vi "GameToIAStateDefensive.vi"(8 "error in (no error)":errorcluster, 11 "Game in":refnum<class "Game.lvclass">) -> (0 "error out":errorcluster, 2 "IA State out":T1={"our_robots"=[], "enemy_robots"=[], "balls"=[], "geometry"={"line_width"=0, "field_length"=0, "field_width"=0, "boundary_width"=0, "referee_width"=0, "goal_width"=0, "goal_depth"=0, "goal_wall_width"=0, "center_circle_radius"=0, "defense_radius"=0, "defense_stretch"=0, "free_kick_from_defense_dist"=0, "penalty_spot_from_field_line_dist"=0, "penalty_line_from_spot_dist"=0}, "IA Judge"={"stage"="", "command"="", "our_goalie_id"=0.0, "enemy_goalie_id"=0.0, "command enum"=enum."Halt", "Time"=enum."Azul", "Point"={"x"=0.0, "y"=0.0}}, "Received Timestamp"=timestamp(0 s since 1904-01-01), "Events"={"Touch"=FALSE, "Ball out"=FALSE, "id touch"=0.0, "Ball out of \nVision"=FALSE, "Ball inside \nGoalie area"=FALSE, "Robot not responding"=FALSE, "Robots responding status"=[1.0, 1.0, 1.0, 1.0, 1.0, 1.0], "Enemy Ball \nPossession"=FALSE, "Pass State"=FALSE, "id end of pass"=0.0, "Kick"=FALSE, "Id ini Possession"=0.0, "Ball Possesion"=FALSE, "Id Possesion"=0.0, "Direct Kick"=FALSE, "2nd Strk Ativo"=FALSE}}, 3 "Game out":refnum<class "Game.lvclass">)   [LabVIEW 2021, in "Game.lvclass"]
uses:
  Game.lvclass
  Vision_class/Old vision/SSL Detection Frame Simple Estimator Cameras VelCmd Folder/Core/AI Input.ctl
  Vision_class/Old vision/Controls/AI Robot.ctl
  Vision_class/Old vision/Controls/Functions Enum.ctl
  Controls/estimatives.ctl
  Vision_class/Old vision/Controls/AttackerStates.ctl
  Vision_class/Old vision/Controls/PathDests.ctl
  Vision_class/Old vision/Controls/PathDest.ctl
  Navigation/VSSNavigation/VSSAttackerStates.ctl
  Robot_class/robotKickToStates.ctl
  Robot_class/roles.ctl
  <vilib>/Analysis/Matrix/Datatypes/RealMatrix.ctl
  Navigation/driveMode.ctl
  Vision_class/Old vision/SSL Detection Frame Simple Estimator Cameras VelCmd Folder/Core/AI Ball.ctl
  Vision_class/Old vision/SSL Detection Frame Simple Estimator Cameras VelCmd Folder/Core/Field Size.ctl
  Vision_class/Old vision/SSL Detection Frame Simple Estimator Cameras VelCmd Folder/Core/AI Judge.ctl
  Communication_class/Paths/MessageAI_State Folder/Intel/Command Enum.ctl
  Vision_class/Old vision/SSL Detection Frame Simple Estimator Cameras VelCmd Folder/Util/Events/Events.ctl
  Game.lvclass/Game.ctl
  Team_class/Team.lvclass/Team.ctl
  Object_class/Object.lvclass/Object.ctl
  Ball_class/Ball.lvclass/Ball.ctl
  Events_class/Events.lvclass/Events.ctl
  Referee_class/Referee.lvclass/Referee.ctl
  Robot_class/Robot.lvclass/Robot.ctl
  Robot_class/Read id.vi
  Object_class/Read x.vi
  Object_class/Read y.vi
  Robot_class/Read orientation.vi
  Robot_class/Read est_v_tang.vi
  Robot_class/Read est_v_norm.vi
  Object_class/Read pos_est_x.vi
  Object_class/Read pos_est_y.vi
  Robot_class/Read dribble.vi
  Robot_class/Read path.vi
  Robot_class/Read path_smooth.vi
  Robot_class/Read dest_x.vi
  Robot_class/Read dest_y.vi
  Robot_class/Read dest_orientation.vi
  Robot_class/Read v_ang.vi
  Robot_class/Read v_norm.vi
  Robot_class/Read v_tang.vi
  Robot_class/Read role.vi
  Read DefensiveTeam.vi
  Read EnemyRef.vi
  Read BallRef.vi
  Read EventsRef.vi
  Read FieldRef.vi
  Read Referee.vi
  Read TimeRef.vi
  Referee_class/Read command_from_referee.vi
  Referee_class/Read command_interpreted.vi
  Events_class/Read ball_inside_enemy_goalie_area.vi
  Events_class/Read ball_inside_our_goalie_area.vi
  Events_class/Read ball_out.vi
  Events_class/Read ball_out_of_vision.vi
  Events_class/Read enemy_ball_possesion.vi
  Events_class/Read id_enemy_ball_possesion.vi
  Events_class/Read id_our_balll_possesion.vi
  Events_class/Read id_touch.vi
  Events_class/Read kick.vi
  Events_class/Read our_balll_possesion.vi
  Events_class/Read touch.vi
  Ball_class/Read v_x.vi
  Ball_class/Read v_y.vi
  Team_class/Read RobotRef.vi
  Ball_class/Ball.lvclass
  D:/RoboIme/horie/SSL_AI/Object_class/Object.lvclass
  Enemy_class/Enemy.lvclass
  D:/RoboIme/horie/SSL_AI/Team_class/Team.lvclass
  Robot_class/Robot.lvclass
  Ally_class/Ally.lvclass
  Events_class/Events.lvclass
  Field_class/Field.lvclass
  Referee_class/Referee.lvclass
  <vilib>/Analysis/Matrix/NI_Matrix.lvlib
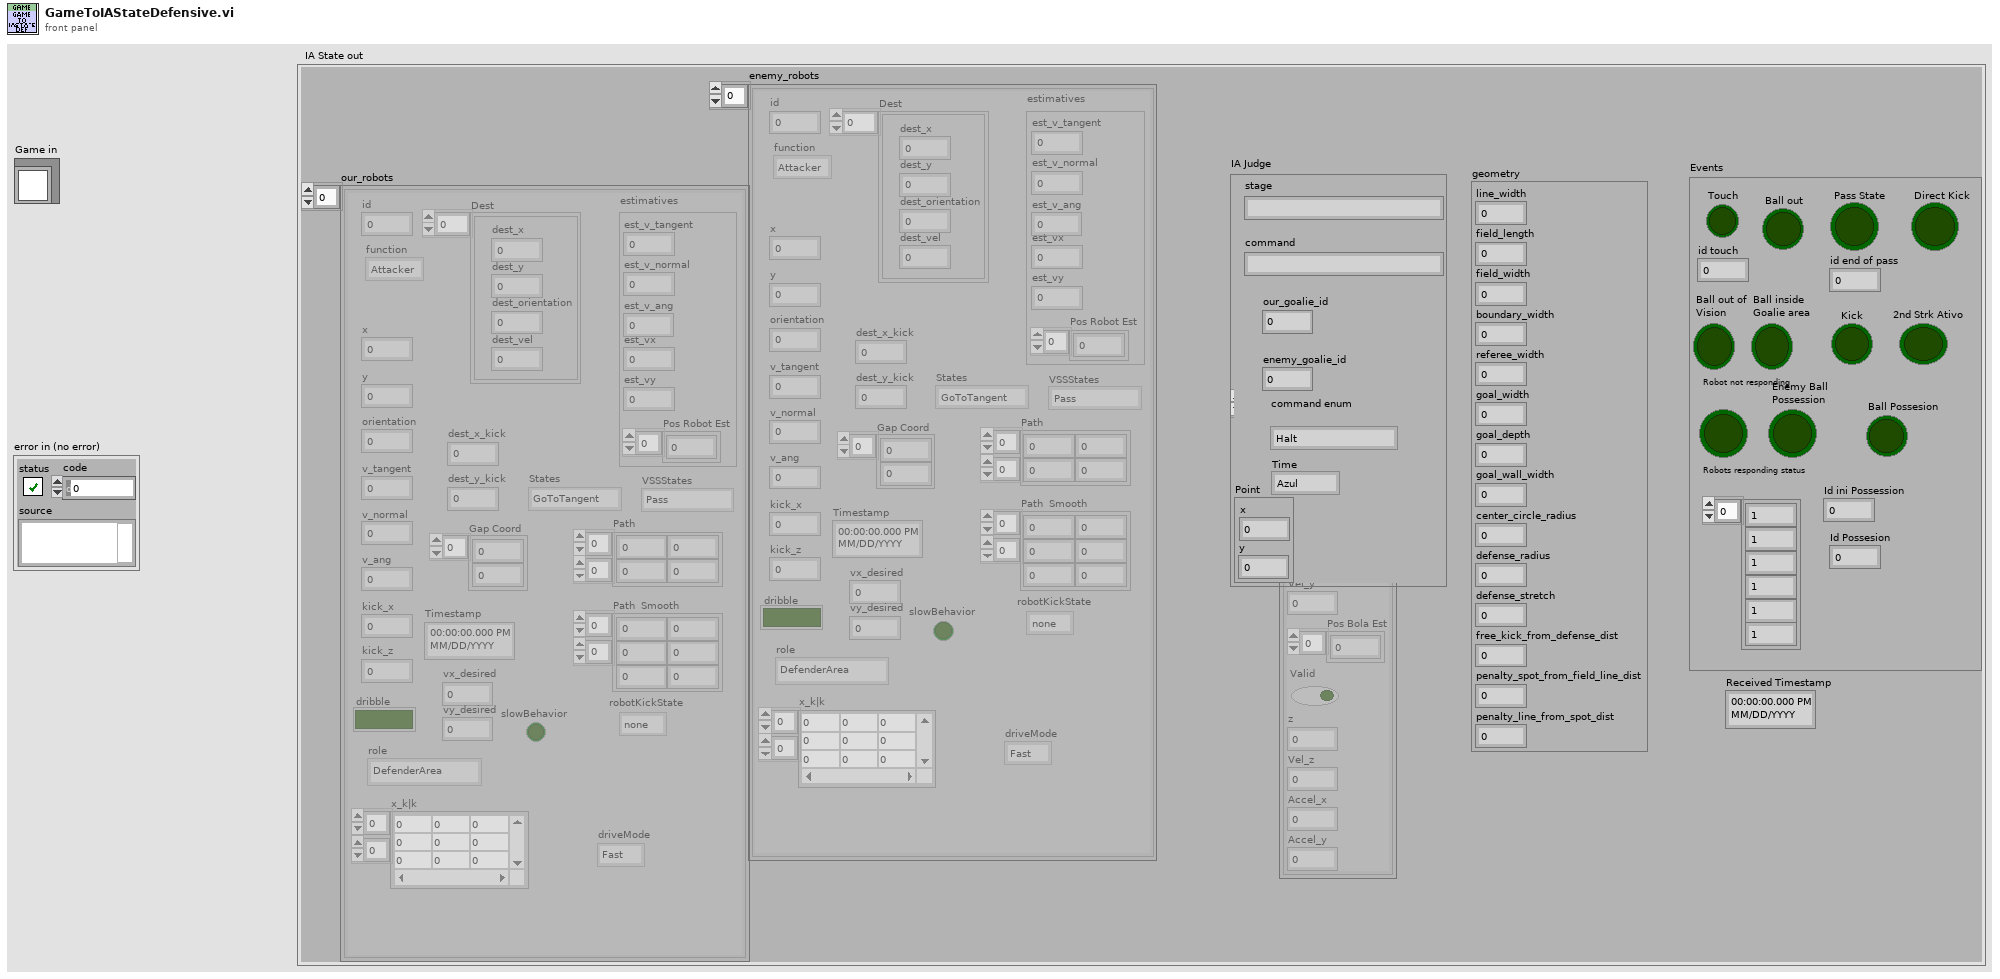
[diagram p1: front panel]
types:
  T1 = typedef "AI Input.ctl" = cluster{"our_robots":T2[], "enemy_robots":T2[], "balls":T13[], "geometry":T14, "IA Judge":T15, "Received Timestamp":timestamp, "Events":T17}
  T2 = typedef "AI Robot.ctl" = cluster{"id":u32, "function":T3, "x":dbl, "y":dbl, "orientation":dbl, "v_tangent":dbl, "v_normal":dbl, "v_ang":dbl, "kick_x":dbl, "kick_z":dbl, "dribble":bool, "Timestamp":timestamp, "estimatives":T4, "dest_x_kick":dbl, "dest_y_kick":dbl, "Gap Coord":dbl[], "States":T5, "Path ":dbl[][], "Path  Smooth":dbl[][], "Dest":T6, "vx_desired":dbl, "vy_desired":dbl, "slowBehavior":bool, "VSSStates":T8, "robotKickState":T9, "role":T10, "x_k|k":T11, "driveMode":T12}
  T3 = typedef "Functions Enum.ctl" = enum16{"2nd Striker", "Attacker", "Goalie", "Defender", "Striker", "Goto 0", "Dummy", "Kicker", "ZigZag 0", "ZigZag 1", "ZigZag 2", "ZigZag 3", "ZigZag 4", "ZigZag 5", "ZigZag 6", "ZigZag 7", "ZigZag 8", ""}
  T4 = typedef "estimatives.ctl" = cluster{"est_v_tangent":dbl, "est_v_normal":dbl, "est_vx":dbl, "est_vy":dbl, "Pos Robot Est":dbl[], "est_v_ang":dbl}
  T5 = typedef "AttackerStates.ctl" = enum16{"Pass", "GoToTangent", "BallGetting", "GoToKick", ""}
  T6 = typedef "PathDests.ctl" = T7[]
  T7 = typedef "PathDest.ctl" = cluster{"dest_x":dbl, "dest_y":dbl, "dest_orientation":dbl, "dest_vel":dbl}
  T8 = typedef "VSSAttackerStates.ctl" = enum16{"Pass", "GoToTangent", "BallGetting", "GoToKick", "Rotate anti-clockwise", "Rotate Clockwise", ""}
  T9 = typedef "robotKickToStates.ctl" = enum16{"shootFromDirect", "avoidCollideBall", "goToBackBall", "none", "walk", "turn", "oldKickToShoot", "oldKickToGoToBackBall", "shoot"}
  T10 = typedef "roles.ctl" = enum16{"SimpleBallPlacement", "BallPlacementAllyPasser", "BallPlacementAllyReceiver", "BallPlacementEnemy", "5Robots5th", "PassBestReceiver", "5Robots4th", "5Robots3rd", "5Robots2nd", "5Robots1st", "PassBestRobot", "WaitPass", "ABCThirdKicker", "ABCFirstKicker", "ABCSecondKicker", "Tabler", "TableFinalizer", "PrepareRollToPassRoller", "PrepareRollToPassReceiver", "SimplePassRoll", "SimplePassRollReceiver", "PenaltyDefense", "PreparePassReceiver 2", "PreparePassReceiver 1", "PassObserver", "Timeout", "Goto", "ZigZag", "None", "BallOutOfField", "DefenderArea", "Duelist", "AttackerStop", "FollowAttacker", "KeeperRole", "KickPenalty", "AttackerAimGoal", "AttackerBlock", "Marker", "Halt", "Shoot", "PassKicker", "PassReceiver", "TestRole", "PenaltyAttacker"}
  T11 = typedef "NI_Matrix.lvlib/RealMatrix.ctl" = dbl[][]
  T12 = typedef "driveMode.ctl" = enum16{"Fast", "SafeDrive"}
  T13 = typedef "AI Ball.ctl" = cluster{"x":dbl, "y":dbl, "timestamp":timestamp, "Vel_x":dbl, "Vel_y":dbl, "Pos Bola Est":dbl[], "Valid":bool, "z":dbl, "Vel_z":dbl, "Accel_x":dbl, "Accel_y":dbl}
  T14 = typedef "Field Size.ctl" = cluster{"line_width":u32, "field_length":u32, "field_width":u32, "boundary_width":u32, "referee_width":u32, "goal_width":u32, "goal_depth":u32, "goal_wall_width":u32, "center_circle_radius":u32, "defense_radius":u32, "defense_stretch":u32, "free_kick_from_defense_dist":u32, "penalty_spot_from_field_line_dist":u32, "penalty_line_from_spot_dist":u32}
  T15 = typedef "AI Judge.ctl" = cluster{"stage":string, "command":string, "our_goalie_id":dbl, "enemy_goalie_id":dbl, "command enum":T16, "Time":enum16{"Azul", "Amarelo"}, "Point":cluster{"x":sgl, "y":sgl}}
  T16 = typedef "Command Enum.ctl" = enum16{"Halt", "Stop", "Force Start", "PKA Normal Start", "Prepare Kickoff Ally", "PKE Normal Start", "Prepare Kickoff Enemy", "Prepare Penalty Ally", "PPA Normal Start", "Prepare Penalty Enemy", "PPE Normal Start", "Direct Free Enemy", "Direct Free Ally", "Indirect Free Enemy", "Indirect Free Ally", "Timeout Enemy", "Timeout Ally", "Goal Enemy", "Goal Ally", "Ball Placement Enemy", "Ball Placement Ally", "Normal Half Time", "Extra Time Break", "Extra Half Time", "None", "Post Game"}
  T17 = typedef "Events.ctl" = cluster{"Touch":bool, "Ball out":bool, "id touch":dbl, "Ball out of \nVision":bool, "Ball inside \nGoalie area":bool, "Robot not responding":bool, "Robots responding status":dbl[], "Enemy Ball \nPossession":bool, "Pass State":bool, "id end of pass":dbl, "Kick":bool, "Id ini Possession":dbl, "Ball Possesion":bool, "Id Possesion":dbl, "Direct Kick":bool, "2nd Strk Ativo":bool}
  T18 = typedef "command_interpreted.ctl" = enum16{"Goal Ally", "Goal Enemy", "Ball Placement Enemy", "Ball Placement Ally", "Normal Half Time", "Extra Time  Break", "Extra Half Time", "None", "Post Game", "PKA Normal Start", "Prepare Kickoff Ally", "PKE Normal Start", "Prepare Kickoff Enemy", "Force Start", "Halt", "Timeout", "Prepare Penalty Ally", "Prepare Penalty Enemy", "PPA NormalStart", "PPE Normal Start", "Indirect Free Ally", "Direct Free Enemy", "Direct Free Ally", "Indirect Free Enemy", "Stop"}
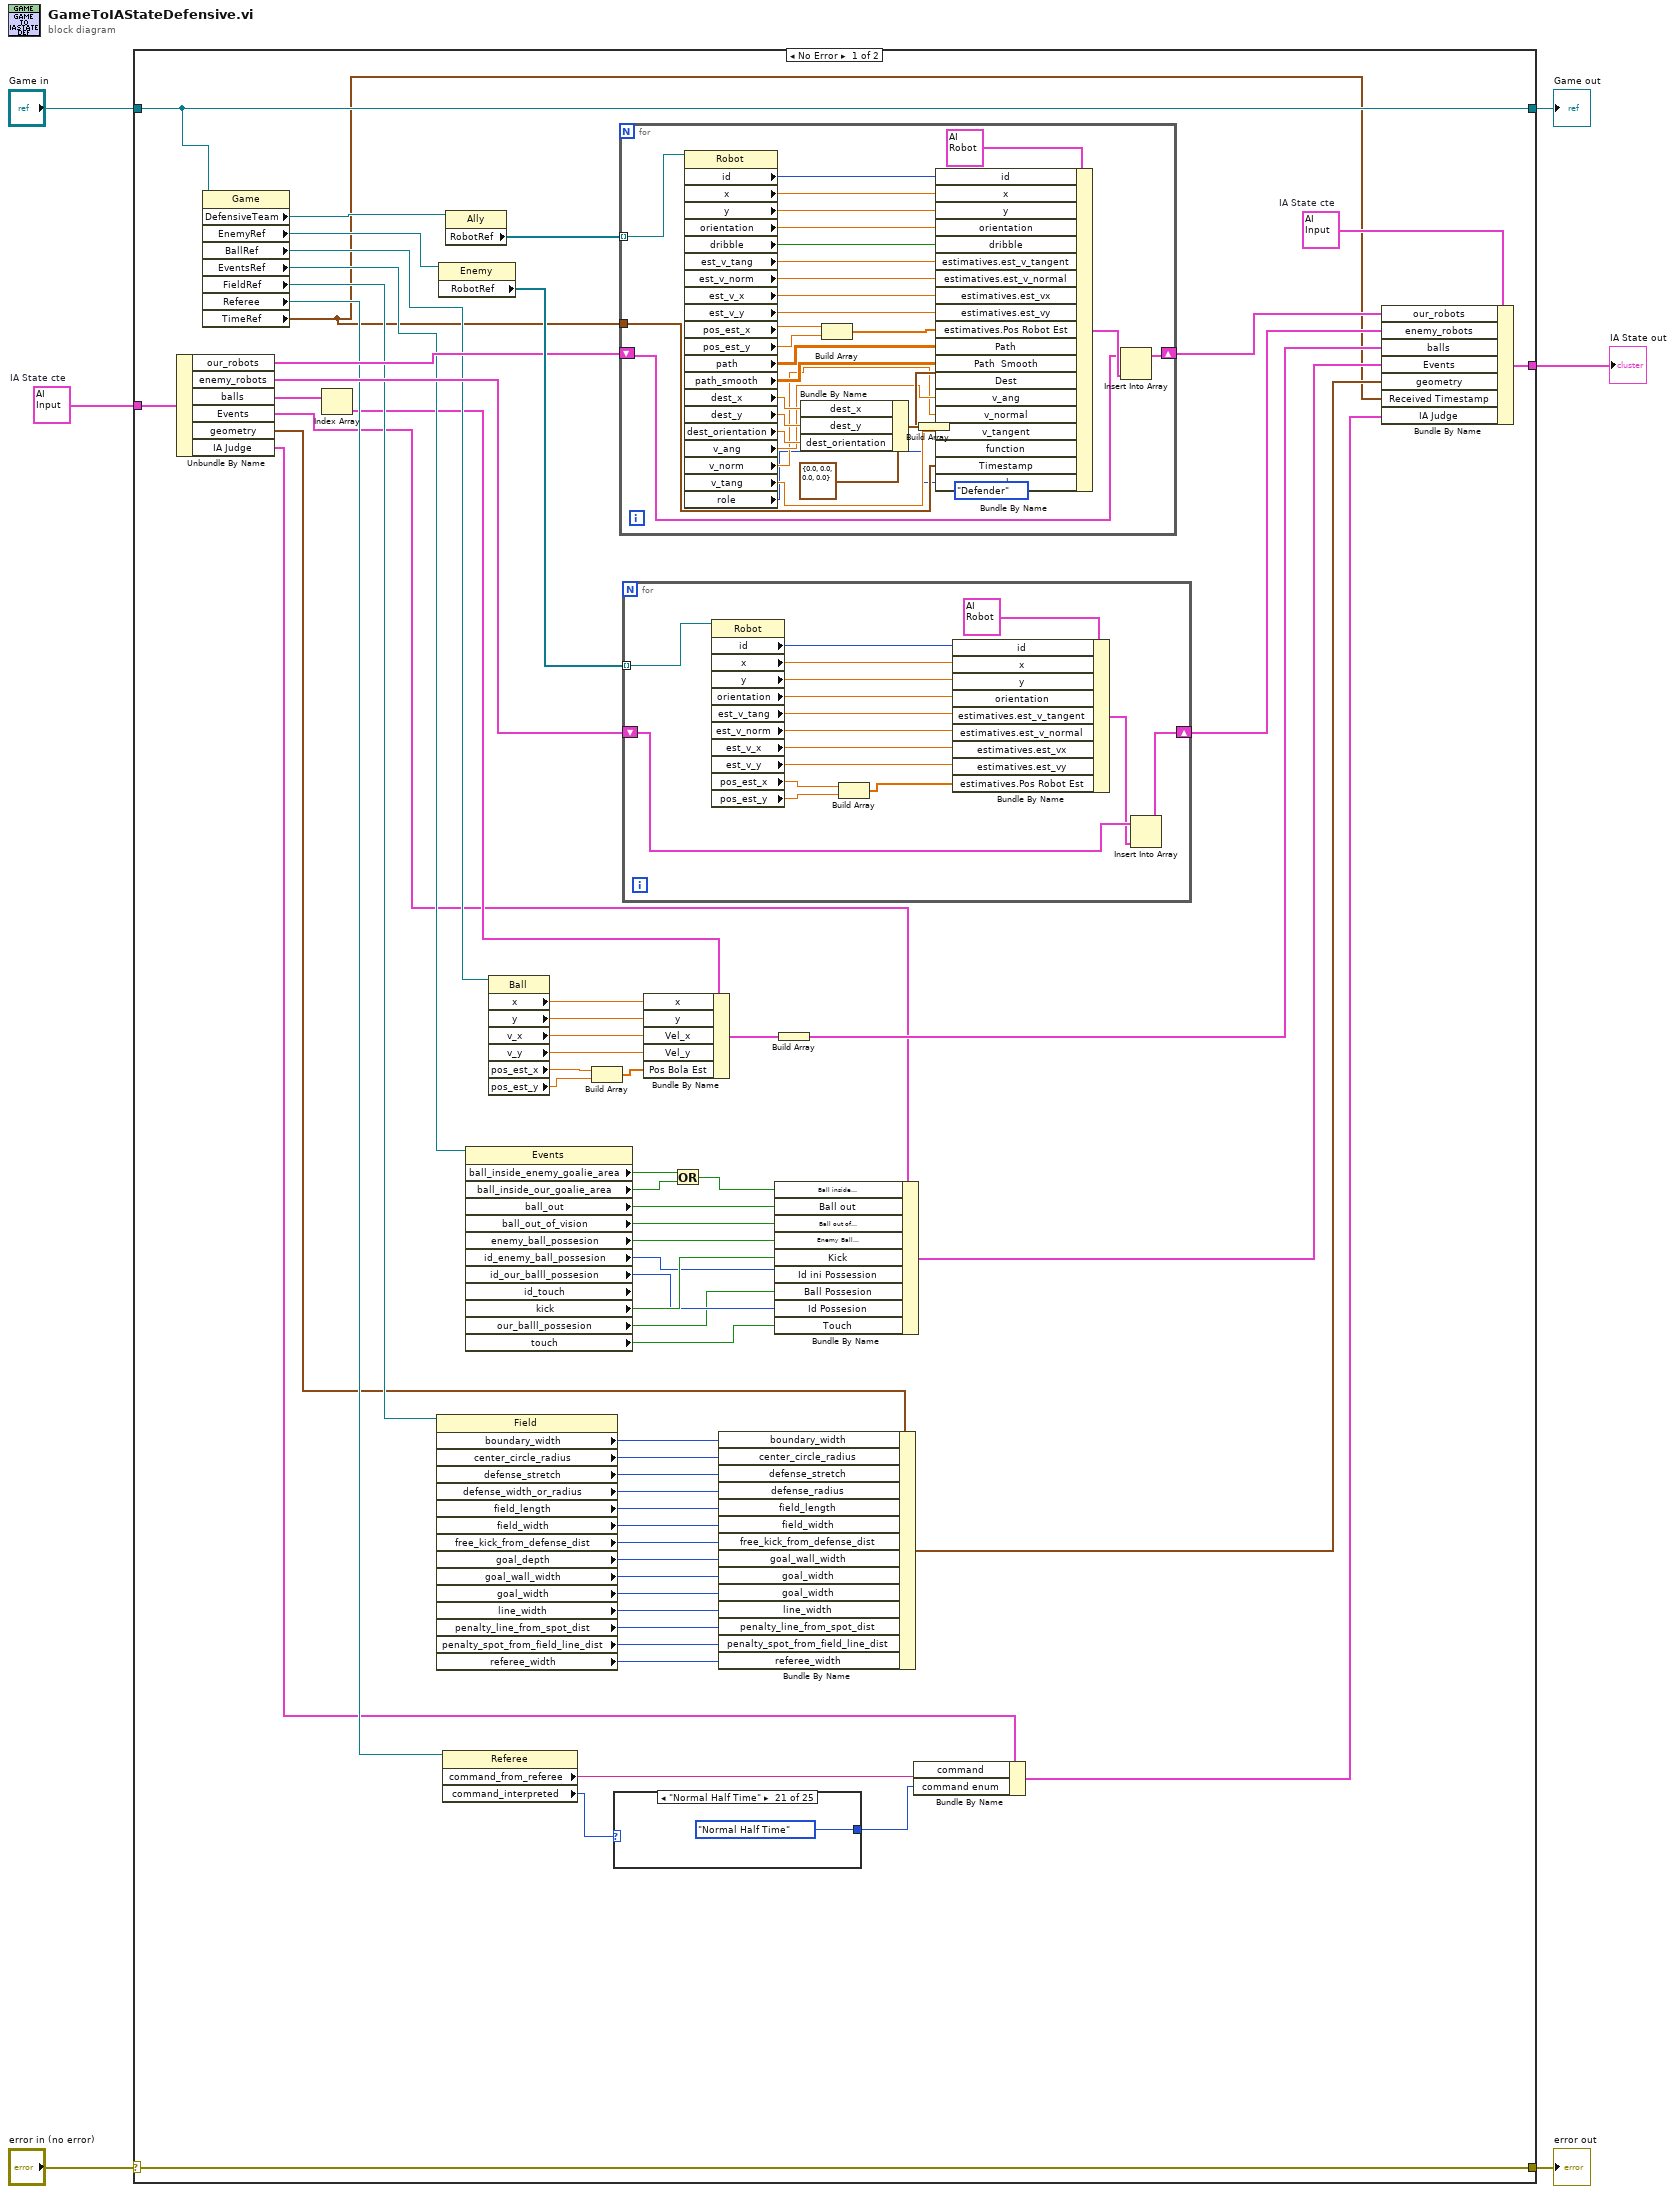
[diagram p0: block diagram]
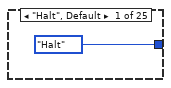
[diagram p2: hidden frame]
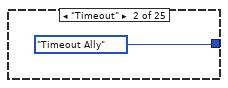
[diagram p3: hidden frame]
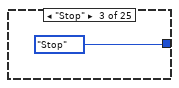
[diagram p4: hidden frame]
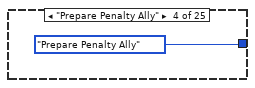
[diagram p5: hidden frame]
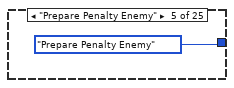
[diagram p6: hidden frame]
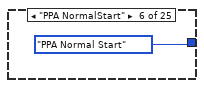
[diagram p7: hidden frame]
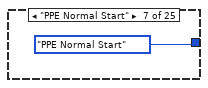
[diagram p8: hidden frame]
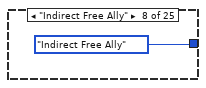
[diagram p9: hidden frame]
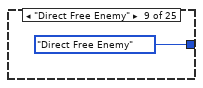
[diagram p10: hidden frame]
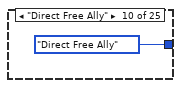
[diagram p11: hidden frame]
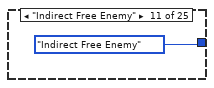
[diagram p12: hidden frame]
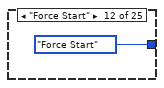
[diagram p13: hidden frame]
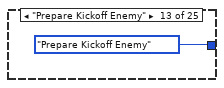
[diagram p14: hidden frame]
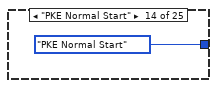
[diagram p15: hidden frame]
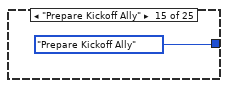
[diagram p16: hidden frame]
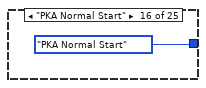
[diagram p17: hidden frame]
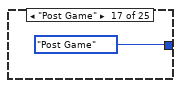
[diagram p18: hidden frame]
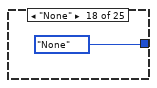
[diagram p19: hidden frame]
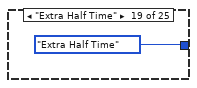
[diagram p20: hidden frame]
diagram:
  w2 = T1 {"our_robots"=[], "enemy_robots"=[], "balls"=[], "geometry"={"line_width"=0, "field_length"=0, "field_width"=0, "boundary_width"=0, "referee_width"=0, "goal_width"=0, "goal_depth"=0, "goal_wall_width"=0, "center_circle_radius"=0, "defense_radius"=0, "defense_stretch"=0, "free_kick_from_defense_dist"=0, "penalty_spot_from_field_line_dist"=0, "penalty_line_from_spot_dist"=0}, "IA Judge"={"stage"="", "command"="", "our_goalie_id"=0.0, "enemy_goalie_id"=0.0, "command enum"=enum."Halt", "Time"=enum."Azul", "Point"={"x"=0.0, "y"=0.0}}, "Received Timestamp"=timestamp(0 s since 1904-01-01), "Events"={"Touch"=FALSE, "Ball out"=FALSE, "id touch"=0.0, "Ball out of \nVision"=FALSE, "Ball inside \nGoalie area"=FALSE, "Robot not responding"=FALSE, "Robots responding status"=[], "Enemy Ball \nPossession"=FALSE, "Pass State"=FALSE, "id end of pass"=0.0, "Kick"=FALSE, "Id ini Possession"=0.0, "Ball Possesion"=FALSE, "Id Possesion"=0.0, "Direct Kick"=FALSE, "2nd Strk Ativo"=FALSE}}  # IA State cte
  n1 = case shown="No Error" "error in (no error)" {
    selector: "error in (no error)" -> [w69 w144]
    tunnel: [w69 w144] -> w5
    tunnel: [w68 w143] -> w3
    tunnel: "Game in" -> [w68 w143]
    tunnel: w2 -> [w63 w142]
    tunnel: [w8 w142] -> w1
    frame No Error {
      w59 = T1 {"our_robots"=[], "enemy_robots"=[], "balls"=[], "geometry"={"line_width"=0, "field_length"=0, "field_width"=0, "boundary_width"=0, "referee_width"=0, "goal_width"=0, "goal_depth"=0, "goal_wall_width"=0, "center_circle_radius"=0, "defense_radius"=0, "defense_stretch"=0, "free_kick_from_defense_dist"=0, "penalty_spot_from_field_line_dist"=0, "penalty_line_from_spot_dist"=0}, "IA Judge"={"stage"="", "command"="", "our_goalie_id"=0.0, "enemy_goalie_id"=0.0, "command enum"=enum."Halt", "Time"=enum."Azul", "Point"={"x"=0.0, "y"=0.0}}, "Received Timestamp"=timestamp(0 s since 1904-01-01), "Events"={"Touch"=FALSE, "Ball out"=FALSE, "id touch"=0.0, "Ball out of \nVision"=FALSE, "Ball inside \nGoalie area"=FALSE, "Robot not responding"=FALSE, "Robots responding status"=[], "Enemy Ball \nPossession"=FALSE, "Pass State"=FALSE, "id end of pass"=0.0, "Kick"=FALSE, "Id ini Possession"=0.0, "Ball Possesion"=FALSE, "Id Possesion"=0.0, "Direct Kick"=FALSE, "2nd Strk Ativo"=FALSE}}  # IA State cte
      n2 = Unbundle By Name(w63) -> ("our_robots"=w62:T2[], "enemy_robots"=w61:T2[], "balls"=w16:T13[], "Events"=w14:T17, "geometry"=w13:T14, "IA Judge"=w12:T15)
      n3 = property class="Game"(reference=w68) -> ("DefensiveTeam"=w67:refnum<class "Ally.lvclass">, "EnemyRef"=w65:refnum<class "Enemy.lvclass">, "BallRef"=w60:refnum<class "Ball.lvclass">, "EventsRef"=w47:refnum<class "Events.lvclass">, "FieldRef"=w34:refnum<class "Field.lvclass">, "Referee"=w18:refnum<class "Referee.lvclass">, "TimeRef"=w7:timestamp)  [unwired: 1 in, 2 out]
      n4 = Index Array(array=w16) -> (element=w15:T13)  [unwired: 1 in]
      n5 = property class="Field"(reference=w34) -> ("boundary_width"=w33:i32, "center_circle_radius"=w32:i32, "defense_stretch"=w31:i32, "defense_width_or_radius"=w30:i32, "field_length"=w29:i32, "field_width"=w28:i32, "free_kick_from_defense_dist"=w27:i32, "goal_depth"=w26:i32, "goal_wall_width"=w25:i32, "goal_width"=w24:i32, "line_width"=w23:i32, "penalty_line_from_spot_dist"=w22:i32, "penalty_spot_from_field_line_dist"=w21:i32, "referee_width"=w20:i32)  [unwired: 1 in, 2 out]
      n6 = property class="Enemy"(reference=w65) -> ("RobotRef"=w64:refnum<class "Robot.lvclass">[])  [unwired: 1 in, 2 out]
      n7 = property class="Referee"(reference=w18) -> ("command_from_referee"=w17:string, "command_interpreted"=w11:T18)  [unwired: 1 in, 2 out]
      n8 = property class="Ally"(reference=w67) -> ("RobotRef"=w66:refnum<class "Robot.lvclass">[])  [unwired: 1 in, 2 out]
      n9 = property class="Events" props=["ball_inside_enemy_goalie_area", "ball_inside_our_goalie_area", "ball_out", "ball_out_of_vision", "enemy_ball_possesion", "id_enemy_ball_possesion", "id_our_balll_possesion", "id_touch", "kick", "our_balll_possesion", "touch"](reference=w47) -> ("ball_inside_enemy_goalie_area"=w45:bool, "ball_inside_our_goalie_area"=w46:bool, "ball_out"=w43:bool, "ball_out_of_vision"=w42:bool, "enemy_ball_possesion"=w41:bool, "id_enemy_ball_possesion"=w39:i32, "id_our_balll_possesion"=w38:i32, "kick"=w40:bool, "our_balll_possesion"=w37:bool, "touch"=w36:bool)  [unwired: 1 in, 3 out]
      n10 = property class="Ball"(reference=w60) -> ("x"=w56:dbl, "y"=w55:dbl, "v_x"=w54:dbl, "v_y"=w53:dbl, "pos_est_x"=w52:dbl, "pos_est_y"=w51:dbl)  [unwired: 1 in, 2 out]
      n11 = Build Array(w52, w51) -> (w50:dbl[])
      n12 = case shown="\"Normal Half Time\"" w11 {
        tunnel: [Command_Enum."Halt" ("command enum") Command_Enum."Timeout Ally" ("command enum") Command_Enum."Stop" ("command enum") Command_Enum."Prepare Penalty Ally" ("command enum") Command_Enum."Prepare Penalty Enemy" ("command enum") Command_Enum."PPA Normal Start" ("command enum") Command_Enum."PPE Normal Start" ("command enum") Command_Enum."Indirect Free Ally" ("command enum") Command_Enum."Direct Free Enemy" ("command enum") Command_Enum."Direct Free Ally" ("command enum") Command_Enum."Indirect Free Enemy" ("command enum") Command_Enum."Force Start" ("command enum") Command_Enum."Prepare Kickoff Enemy" ("command enum") Command_Enum."PKE Normal Start" ("command enum") Command_Enum."Prepare Kickoff Ally" ("command enum") Command_Enum."PKA Normal Start" ("command enum") Command_Enum."Post Game" ("command enum") Command_Enum."None" ("command enum") Command_Enum."Extra Half Time" ("command enum") Command_Enum."Extra Time Break" ("command enum") Command_Enum."Normal Half Time" ("command enum") Command_Enum."Ball Placement Ally" ("command enum") Command_Enum."Ball Placement Enemy" ("command enum") Command_Enum."Goal Enemy" ("command enum") Command_Enum."Goal Ally" ("command enum")] -> w10
        frame "Halt", Default {
        }
        frame "Timeout" {
        }
        frame "Stop" {
        }
        frame "Prepare Penalty Ally" {
        }
        frame "Prepare Penalty Enemy" {
        }
        frame "PPA NormalStart" {
        }
        frame "PPE Normal Start" {
        }
        frame "Indirect Free Ally" {
        }
        frame "Direct Free Enemy" {
        }
        frame "Direct Free Ally" {
        }
        frame "Indirect Free Enemy" {
        }
        frame "Force Start" {
        }
        frame "Prepare Kickoff Enemy" {
        }
        frame "PKE Normal Start" {
        }
        frame "Prepare Kickoff Ally" {
        }
        frame "PKA Normal Start" {
        }
        frame "Post Game" {
        }
        frame "None" {
        }
        frame "Extra Half Time" {
        }
        frame "Extra Time  Break" {
        }
        frame "Normal Half Time" {
        }
        frame "Ball Placement Ally" {
        }
        frame "Ball Placement Enemy" {
        }
        frame "Goal Enemy" {
        }
        frame "Goal Ally" {
        }
      }
      n13 = for {
        tunnel: w66 -> [w121] mode=indexing
        shift-right: [w122] -> w58
        shift-left: w62 -> [w123]
        tunnel: w7 -> [w96]
        n14 = property class="Robot"(reference=w121) -> ("id"=w120:i32, "x"=w119:dbl, "y"=w118:dbl, "orientation"=w117:dbl, "dribble"=w116:bool, "est_v_tang"=w115:dbl, "est_v_norm"=w114:dbl, "est_v_x"=w113:dbl, "est_v_y"=w112:dbl, "pos_est_x"=w111:dbl, "pos_est_y"=w110:dbl, "path"=w108:dbl[][], "path_smooth"=w107:dbl[][], "dest_x"=w106:dbl, "dest_y"=w105:dbl, "dest_orientation"=w104:dbl, "v_ang"=w100:dbl, "v_norm"=w99:dbl, "v_tang"=w98:dbl, "role"=w95:T10)  [unwired: 1 in, 2 out]
        n15 = Bundle By Name(cluster=T7 {"dest_x"=0.0, "dest_y"=0.0, "dest_orientation"=0.0, "dest_vel"=0.0} ("element"), "dest_x"=w106, "dest_y"=w105, "dest_orientation"=w104) -> (w102:T7)
        n16 = Build Array(w111, w110) -> (w109:dbl[])
        n17 = Build Array(w102) -> (w101:T7[])
        n18 = Bundle By Name(cluster=T2 {"id"=0, "function"=enum."Attacker", "x"=0.0, "y"=0.0, "orientation"=0.0, "v_tangent"=0.0, "v_normal"=0.0, "v_ang"=0.0, "kick_x"=0.0, "kick_z"=0.0, "dribble"=FALSE, "Timestamp"=timestamp(0 s since 1904-01-01), "estimatives"={"est_v_tangent"=0.0, "est_v_normal"=0.0, "est_vx"=0.0, "est_vy"=0.0, "Pos Robot Est"=[], "est_v_ang"=0.0}, "dest_x_kick"=0.0, "dest_y_kick"=0.0, "Gap Coord"=[], "States"=enum."GoToTangent", "Path "=[], "Path  Smooth"=[], "Dest"=[], "vx_desired"=0.0, "vy_desired"=0.0, "slowBehavior"=FALSE, "VSSStates"=enum."Pass", "robotKickState"=enum."none", "role"=enum."DefenderArea", "x_k|k"=[], "driveMode"=enum."Fast"} ("Robot"), "id"=w120, "x"=w119, "y"=w118, "orientation"=w117, "dribble"=w116, "estimatives.est_v_tangent"=w115, "estimatives.est_v_normal"=w114, "estimatives.est_vx"=w113, "estimatives.est_vy"=w112, "estimatives.Pos Robot Est"=w109, "Path"=w108, "Path  Smooth"=w107, "Dest"=w101, "v_ang"=w100, "v_normal"=w99, "v_tangent"=w98, "function"=Functions_Enum."Defender", "Timestamp"=w96, "role"=w95) -> (w124:T2)
        n19 = Insert Into Array(array=w123, new element=w124) -> (w122:T2[])  [unwired: 1 in]
      }
      n20 = for {
        tunnel: w64 -> [w136] mode=indexing
        shift-right: [w126] -> w57
        shift-left: w61 -> [w135]
        n21 = property class="Robot"(reference=w136) -> ("id"=w138:i32, "x"=w139:dbl, "y"=w140:dbl, "orientation"=w141:dbl, "est_v_tang"=w134:dbl, "est_v_norm"=w133:dbl, "est_v_x"=w132:dbl, "est_v_y"=w131:dbl, "pos_est_x"=w130:dbl, "pos_est_y"=w129:dbl)  [unwired: 1 in, 2 out]
        n22 = Build Array(w130, w129) -> (w128:dbl[])
        n23 = Bundle By Name(cluster=T2 {"id"=0, "function"=enum."Attacker", "x"=0.0, "y"=0.0, "orientation"=0.0, "v_tangent"=0.0, "v_normal"=0.0, "v_ang"=0.0, "kick_x"=0.0, "kick_z"=0.0, "dribble"=FALSE, "Timestamp"=timestamp(0 s since 1904-01-01), "estimatives"={"est_v_tangent"=0.0, "est_v_normal"=0.0, "est_vx"=0.0, "est_vy"=0.0, "Pos Robot Est"=[], "est_v_ang"=0.0}, "dest_x_kick"=0.0, "dest_y_kick"=0.0, "Gap Coord"=[], "States"=enum."GoToTangent", "Path "=[], "Path  Smooth"=[], "Dest"=[], "vx_desired"=0.0, "vy_desired"=0.0, "slowBehavior"=FALSE, "VSSStates"=enum."Pass", "robotKickState"=enum."none", "role"=enum."DefenderArea", "x_k|k"=[], "driveMode"=enum."Fast"} ("Robot"), "id"=w138, "x"=w139, "y"=w140, "orientation"=w141, "estimatives.est_v_tangent"=w134, "estimatives.est_v_normal"=w133, "estimatives.est_vx"=w132, "estimatives.est_vy"=w131, "estimatives.Pos Robot Est"=w128) -> (w127:T2)
        n24 = Insert Into Array(array=w135, new element=w127) -> (w126:T2[])  [unwired: 1 in]
      }
      n25 = Bundle By Name(cluster=w15, "x"=w56, "y"=w55, "Vel_x"=w54, "Vel_y"=w53, "Pos Bola Est"=w50) -> (w49:T13)
      n26 = Or(x=w45, y=w46) -> (x .or. y?=w44:bool)
      n27 = Bundle By Name(cluster=w13, "boundary_width"=w33, "center_circle_radius"=w32, "defense_stretch"=w31, "defense_radius"=w30, "field_length"=w29, "field_width"=w28, "free_kick_from_defense_dist"=w27, "goal_wall_width"=w26, "goal_width"=w25, "goal_width"=w24, "line_width"=w23, "penalty_line_from_spot_dist"=w22, "penalty_spot_from_field_line_dist"=w21, "referee_width"=w20) -> (w19:T14)
      n28 = Bundle By Name(cluster=w14, "Ball inside \nGoalie area"=w44, "Ball out"=w43, "Ball out of \nVision"=w42, "Enemy Ball \nPossession"=w41, "Kick"=w40, "Id ini Possession"=w39, "Ball Possesion"=w37, "Id Possesion"=w38, "Touch"=w36) -> (w35:T17)
      n29 = Build Array(w49) -> (w48:T13[])
      n30 = Bundle By Name(cluster=w12, "command"=w17, "command enum"=w10) -> (w9:T15)
      n31 = Bundle By Name(cluster=w59, "our_robots"=w58, "enemy_robots"=w57, "balls"=w48, "Events"=w35, "geometry"=w19, "Received Timestamp"=w7, "IA Judge"=w9) -> (w8:T1)
    }
    frame Error {
    }
  }
  "error out" <- w5
  "Game out" <- w3
  "IA State out" <- w1
